vi "GFITS_TryCreateImage.vi"(0 "rootname":string, 1 "logfile":path, 2 "newimsep":string="-", 5 "datatype":i32, 7 "hdutype":i32, 9 "amplifiers":u64, 11 "error in (no error)":errorcluster, 12 "multiple extensions":bool, 13 "retries on error":i16=20, 14 "totkeys":i32) -> (4 "imname out":string, 8 "return value":u64, 15 "error out":errorcluster)   [LabVIEW 2016]
uses:
  DBSHAND/private/vis/DatabaseHand_Element_Get(string).vi
  DBSHAND/private/vis/DatabaseHand_Element_Get(bool).vi
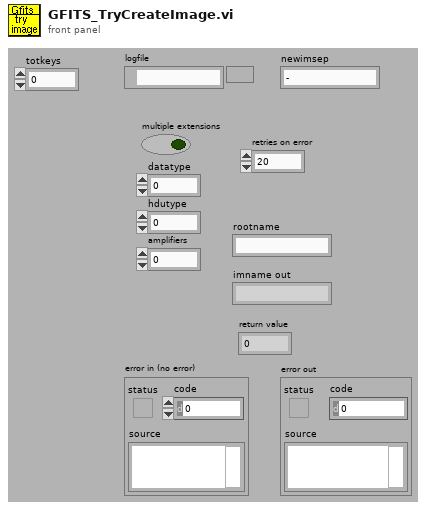
[diagram p1: front panel]
types:
  T1 = typedef "DatabaseHand_RefNum.ctl" = refnum<vi>
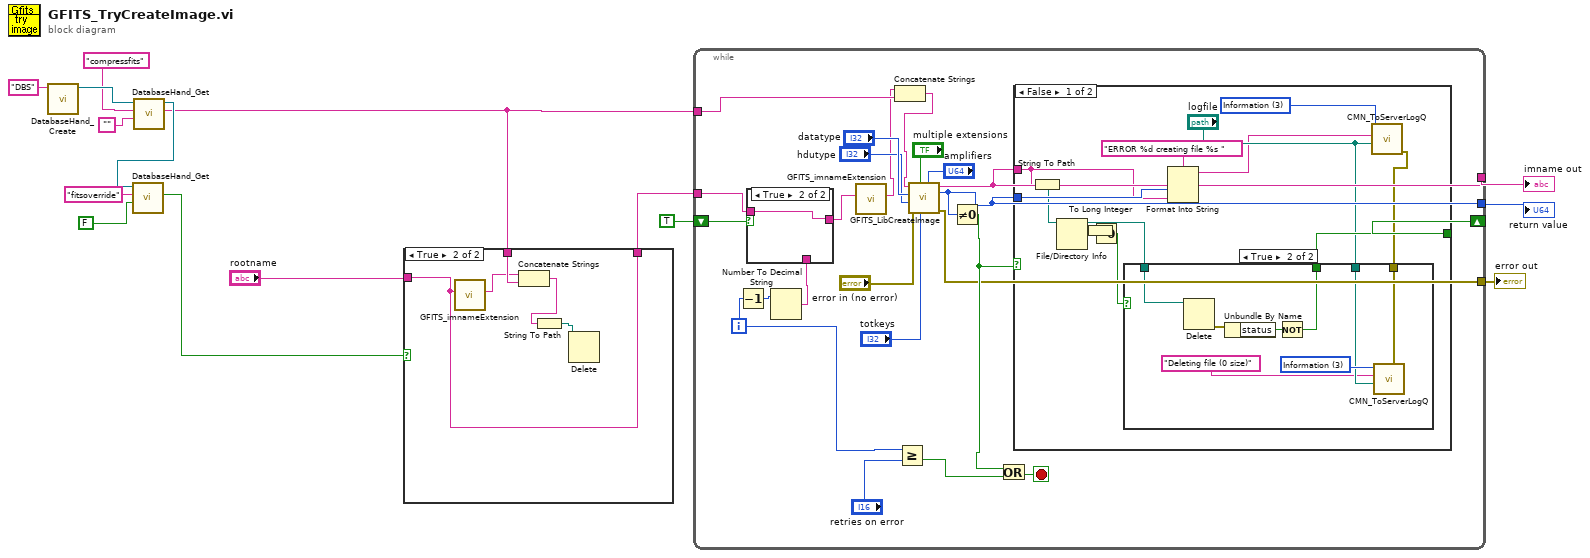
[diagram p0: block diagram]
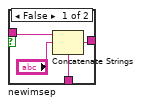
[diagram p5: hidden frame]
diagram:
  n1 = call "DatabaseHand_Create.vi"("Name"="DBS") -> ("Database RefNum out"=w10:T1)  [unwired: 1 in, 9 out]
  n2 = call-poly "DatabaseHand_Get.vi"("default value"="", "name"="compressfits", "Database RefNum in"=w10) -> ("value"=w2:string, "Database RefNum out"=w7:T1)  [unwired: 2 in, 5 out]
  n3 = call-poly "DatabaseHand_Get.vi"("default value"=FALSE, "name"="fitsoverride", "Database RefNum in"=w7) -> ("value"=w5:bool)  [unwired: 2 in, 6 out]
  n4 = case shown="True" w5 {
    tunnel: "rootname" -> [w16 w17]
    tunnel: [w16 w17] -> w3
    tunnel: w2 -> [_ w21]
    frame False {
    }
    frame True {
      n5 = call "GFITS_imnameExtension.vi"("imname in"=w17) -> ("imname out"=w20:string)  [unwired: 9 out]
      n6 = Concatenate Strings(w20, w21) -> (w19:string)
      n7 = String To Path(string=w19) -> (path=w18:path)
      n8 = Delete(path (use dialog)=w18) -> ()  [unwired: 1 in, 6 out]
    }
  }
  n9 = while {
    tunnel: [w29] -> w13
    tunnel: [w30] -> w14
    shift-right: [w28] -> _
    shift-left: TRUE -> [w43]
    tunnel: w3 -> [w38]
    tunnel: [w26] -> w12
    tunnel: w2 -> [w24]
    i -> [w33]
    stop <- w36 stop-if-true
    n10 = Decrement(x=w33) -> (x-1=w34:i32)
    n11 = Number To Decimal String(number=w34) -> (decimal integer string=w44:string)  [unwired: 1 out]
    n12 = case shown="True" w43 {
      tunnel: w44 -> [w71 _]
      tunnel: w38 -> [w70 w72]
      tunnel: [w69 w72] -> w39
      frame False {
        n13 = Concatenate Strings(w70, "newimsep", w71) -> (w69:string)
      }
      frame True {
      }
    }
    n14 = call "GFITS_imnameExtension.vi"("imname in"=w39) -> ("imname out"=w23:string)  [unwired: 9 out]
    n15 = Concatenate Strings(w23, w24) -> (w25:string)
    n16 = Greater Or Equal?(x=w33, y="retries on error") -> (x >= y?=w32:bool)
    n17 = call "GFITS_LibCreateImage.vi"("amplifiers"="amplifiers", "totkeys"="totkeys", "multiple extensions"="multiple extensions", "error in (no error)"="error in (no error)", "hdutype"="hdutype", "datatype"="datatype", "imname"=w25) -> ("error out"=w26:errorcluster, "return value"=w29:u64, "imname out"=w30:string)  [unwired: 2 out]
    n18 = Not Equal To 0?(x=w29) -> (x != 0?=w31:bool)
    n19 = Or(x=w31, y=w32) -> (x .or. y?=w36:bool)
    n20 = case shown="False" w31 {
      selector: w31 -> [_ w67]
      tunnel: w30 -> [w55 _]
      tunnel: w29 -> [w57 _]
      tunnel: [w50 w67] -> w28
      frame False {
        w56 = u16 3 items=["command", "imediateReply", "Callback Reply", "Information", "none"] ("type")
        n21 = String To Path(string=w55) -> (path=w54:path)
        n22 = File/Directory Info(path=w54) -> (path out=w52:path, size=w45:i64)  [unwired: 1 in, 5 out]
        n23 = To Long Integer(number=w45) -> (32bit integer=w53:i32)
        n24 = Equal To 0?(x=w53) -> (x = 0?=w51:bool)
        n25 = Format Into String(format string="ERROR %d creating file %s " ("string"), w57, w55) -> (resulting string=w47:string)  [unwired: 2 in, 1 out]
        n26 = call "CMN_ToServerLogQ.vi"("file"="logfile", "string"=w47, "type"=w56) -> ("error out"=w49:errorcluster)  [unwired: 3 in, 4 out]
        n27 = case shown="True" w51 {
          selector: w51 -> [w58 _]
          tunnel: w52 -> [_ w66]
          tunnel: [w58 w63] -> w50
          tunnel: w49 -> [_ w61]
          tunnel: "logfile" -> [_ w60]
          frame False {
          }
          frame True {
            w62 = u16 3 items=["command", "imediateReply", "Callback Reply", "Information", "none"] ("type")
            n28 = Delete(path (use dialog)=w66) -> (error out=w65:errorcluster)  [unwired: 1 in, 5 out]
            n29 = Unbundle By Name(w65) -> ("status"=w64:bool)
            n30 = Not(x=w64) -> (.not. x?=w63:bool)
            n31 = call "CMN_ToServerLogQ.vi"("error in (no error)"=w61, "file"=w60, "string"="Deleting file (0 size)" ("format string"), "type"=w62) -> ()  [unwired: 2 in, 5 out]
          }
        }
      }
      frame True {
      }
    }
  }
  "imname out" <- w14
  "return value" <- w13
  "error out" <- w12
